vi "ResetCounter.vi"(1 "Reset":bool, 2 "Increment":bool) -> (0 "x+1":u16)   [LabVIEW 2019]
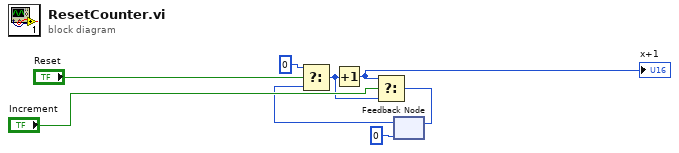
[diagram p0: block diagram]
diagram:
  n1 = feedback #1(u16 0 ("t")) -> (w2:u16)
  n2 = Select(t=u16 0, s="Reset", f=w2) -> (s? t:f=w4:u16)
  n3 = Increment(x=w4) -> (x+1=w6:u16)
  "x+1" <- w6
  n4 = Select(t=w6, s="Increment", f=w4) -> (s? t:f=w3:u16)
  n5 = feedback-in #1(w3) -> ()
